vi "Retroespalhamento.vi"() -> ()   [LabVIEW 2019]
uses:
  <vilib>/Analysis/4window.llb/windowTd.ctl
  <vilib>/Analysis/baseanly.llb/Mean (DBL).vi
  <vilib>/Waveform/WDTOps.llb/WDT Number of Waveform Samples DBL.vi
  <vilib>/Waveform/WDTOps.llb/WDT Get Waveform Subset DBL (LV80).vi
  Agilent 6000 Series/Public/Data/Read Single Waveform.vi
  <vilib>/measure/maspectr.llb/FFT Power Spectral Density for 1 Chan.vi
  Instance           2 25Saved   Retroespalhamento .vi
  Instance           4 25Saved   Retroespalhamento .vi
  Instance           3 25Saved   Retroespalhamento .vi
  <vilib>/Analysis/NI_AALPro.lvlib
  Agilent 2000 3000 X-Series/Agilent 2000 3000 X-Series.lvlib
  Agilent 6000 Series/Agilent 6000 Series.lvlib
  <vilib>/measure/NI_MABase.lvlib
  <vilib>/gmath/NI_Gmath.lvlib
  <vilib>/measure/NI_MAPro.lvlib
  <vilib>/Analysis/NI_AALBase.lvlib
panel:
  in  "Freq":dbl
  in  "N of Sample":dbl
  out "Valores do Arquivo TXT":i32[](array[numeric])
  out "output cluster":T1
  out "dfnovo":dbl
  out "FFT1":waveform(dbl)(graph)
  out "FFT2":waveform(dbl)(graph)
  out "df 2":dbl
  out "Espectro novo":dbl[](array[numeric]) format="%_6g"
  in  "Observações":string
  in  "Jump Button":bool
  in  "Save Button":bool
  out "refnum out":refnum<file>
  in  "Repetição":u16(ring) items=["Repetição 1", "Repetição 2", "Repetição 3", "Repetição 4"]
  out "Tabela de Resultados":string[][](table)=[["Repetição ", "AIB", "FSAB", "TSAB"], ["1", "0", "0", "0"], ["2", "0", "0", "0"], ["3", "0", "0", "0"], ["4", "0", "0", "0"]]
  out "TSAB":dbl format="%#_3g"
  in  "Play Button 2":bool
  out "TSAB":dynamicdata(graph)
  out "AIB's":dbl[](array[numeric])
  out "Freq. central":dbl format="%#_3g"
  out "FSAB":dbl format="%#_3g"
  out "size(s)":i32
  out "AIB":dbl format="%#_5g"
  out "Fmax":dbl format="%#_3g"
  out "Fmin":dbl format="%#_3g"
  out "df":dbl
  out "dt":dbl
  in  "Filename":path=path "test.lvm"
  out "FSAB":dynamicdata(graph)
  out "ABTF":waveform(dbl)(graph)
  out "ABTF":dbl[](array[numeric])
  in  "Play Button":bool
  in  "method 4":u16(ring) items=["Least Square", "Least Absolute Residual", "Bisquare"]
  out "Espectro osso":dbl[](array[numeric])
  in  "Captura 2":bool
  in  "Captura":bool
  in  "Parar":bool
  out "Espectro referência":dbl[](array[numeric])
  in  "Quantidade de Capturas":dbl
  out "Waveform com osso":waveform(dbl)(graph)
  in  "method 3":u16(ring) items=["Least Square", "Least Absolute Residual", "Bisquare"]
  in  "Signal Conditioning?":bool
  out "Waveform Referência":waveform(dbl)(graph)
  in  "Maximum Time (10000 ms)":u32
  in  "VISA":refnum<visa-resource-name>
  in  "Channel":u16(ring) items=["Channel 1", "Channel 2", "Channel 3", "Channel 4"]
  in  "Osciloscópio":u16(ring)=4 items=["DSO 3024A", "DSO 6032A", "Simulation", "Data PEB", "Data Labus", "Choose a Scope"]
  # "Resultados (Résultats)"
  # "Osso (Os)"
  # "Cálculos (Calculs)"
  # "Referência (Référence)"
  # "Configurações"
  # "Osciloscópio"
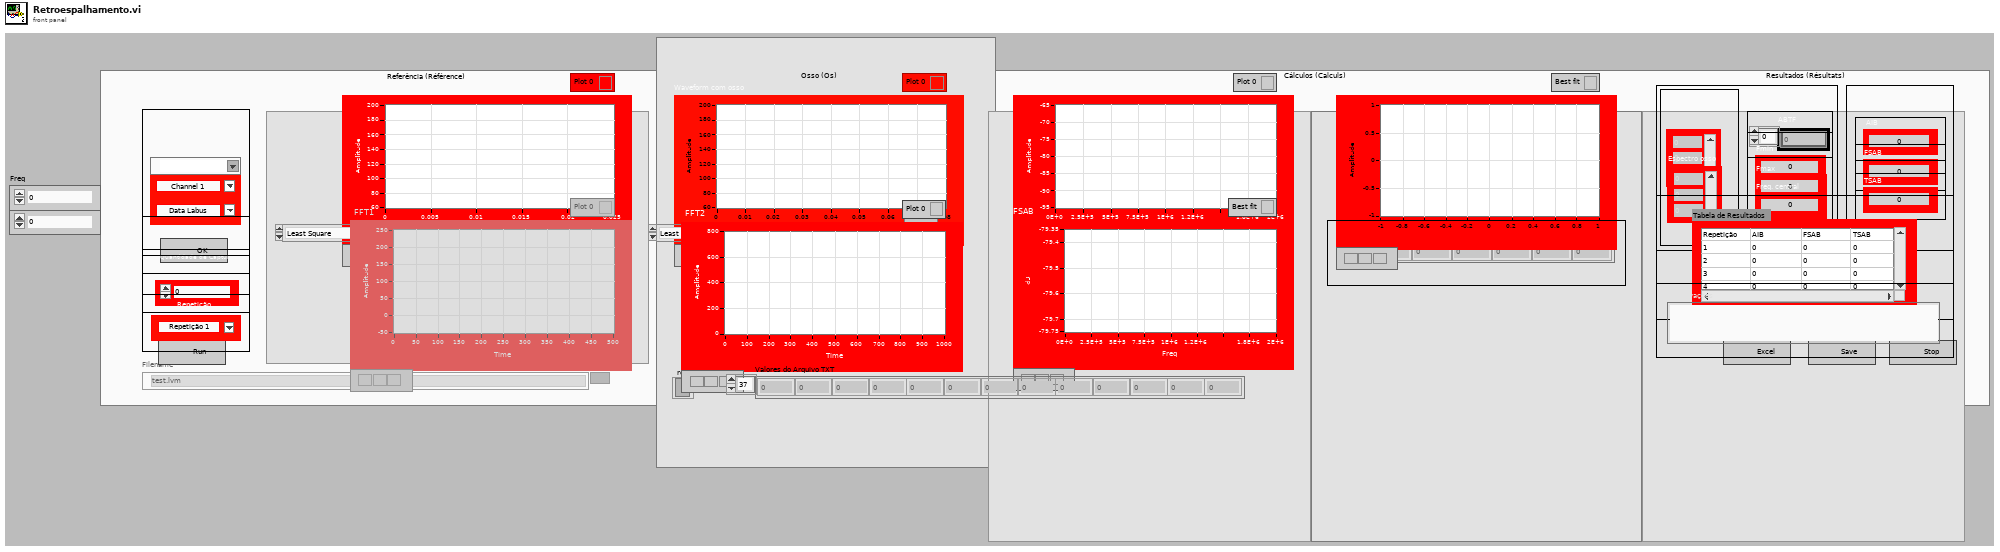
[diagram p1: front panel]
types:
  T1 = cluster{"Waveform Referência":waveform(dbl), "Waveform com osso":waveform(dbl), " FFT1":waveform(dbl), " FFT2":waveform(dbl), "FSAB":dynamicdata, " ABTF":waveform(dbl), "TSAB":dynamicdata, "Tabela de Resultados":string[][], "AIB":dbl, "Fmin":dbl, "Fmax":dbl, "AIB's":dbl[], "TSAB":dbl, "FSAB":dbl, "Observações":string}
  T2 = enum16{"Sine Wave", "Triangle Wave", "Square Wave", "Sawtooth Wave"}
  T3 = enum8{"Enabled", "Disabled", "Disabled and Grayed Out"}
  T4 = typedef "NI_AALPro.lvlib/windowTd.ctl" = u32
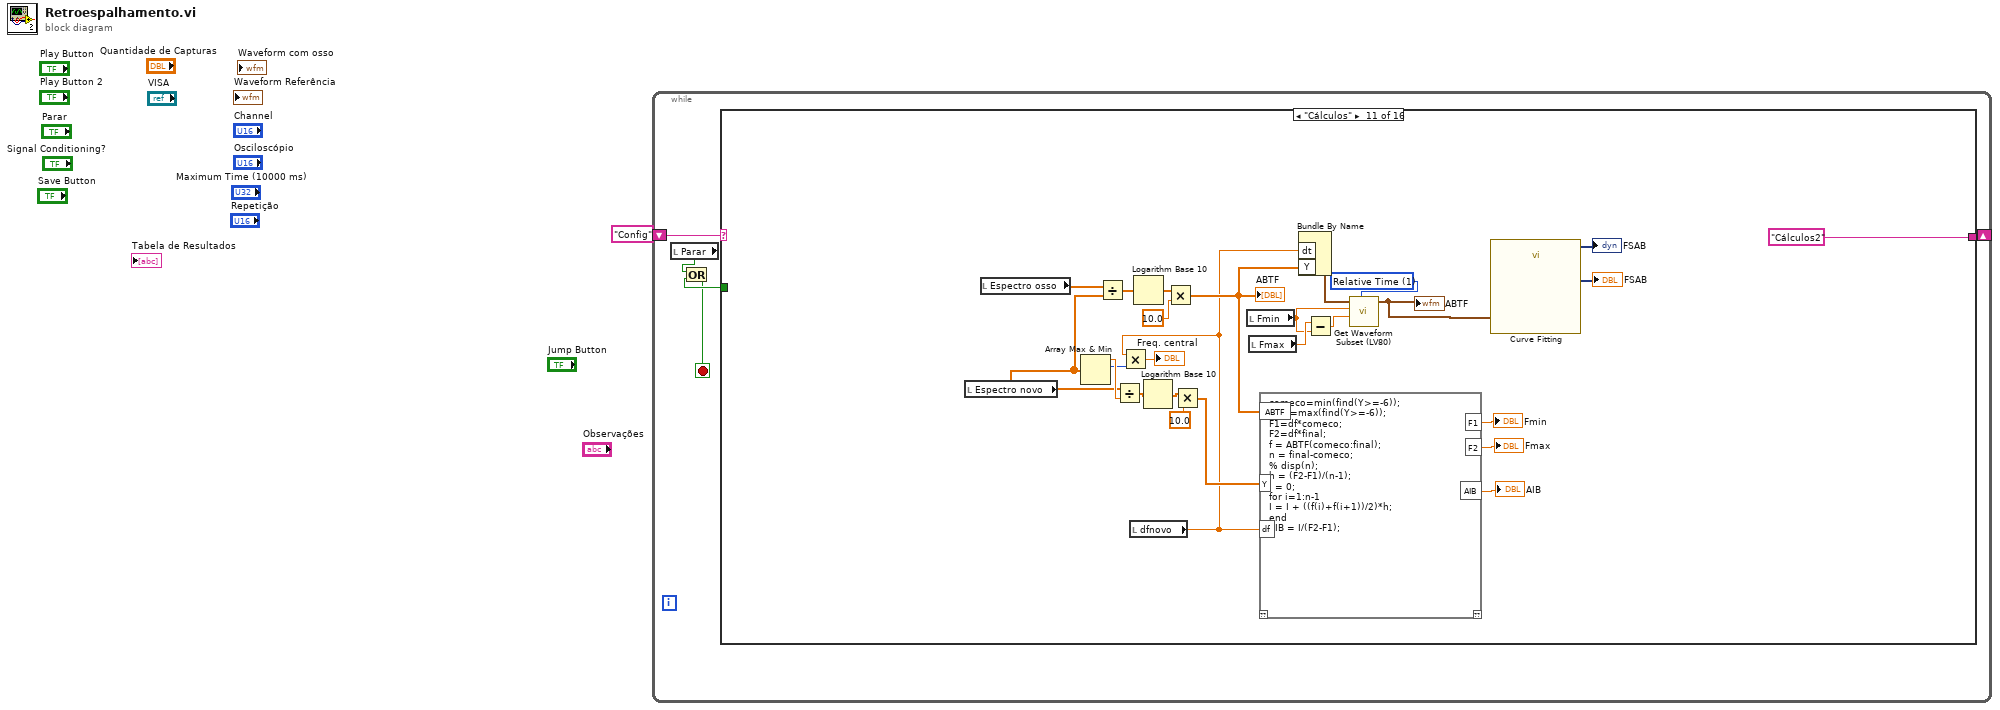
[diagram p0: block diagram]
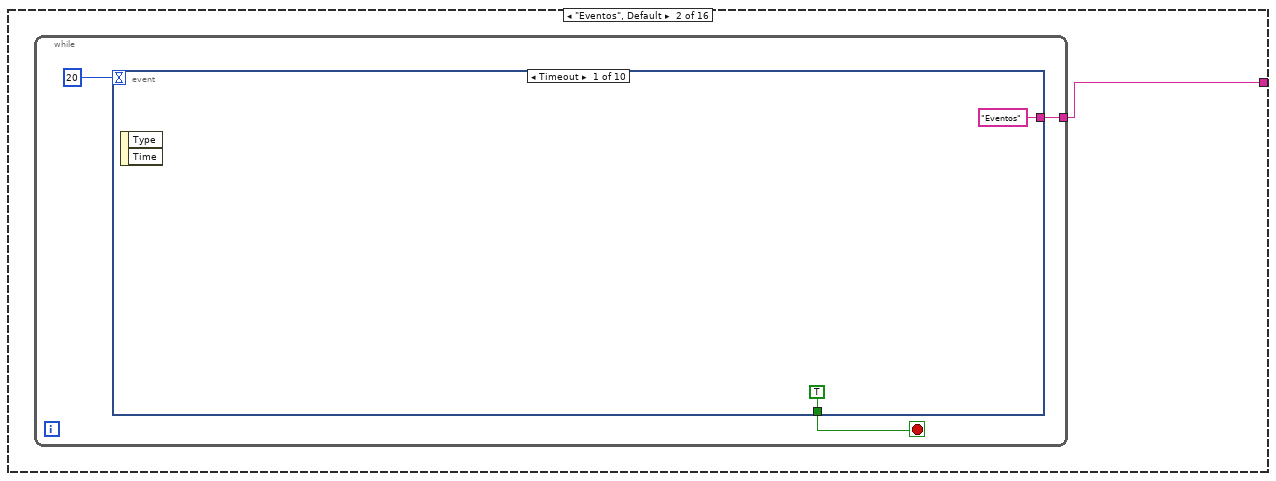
[diagram p3: hidden frame]
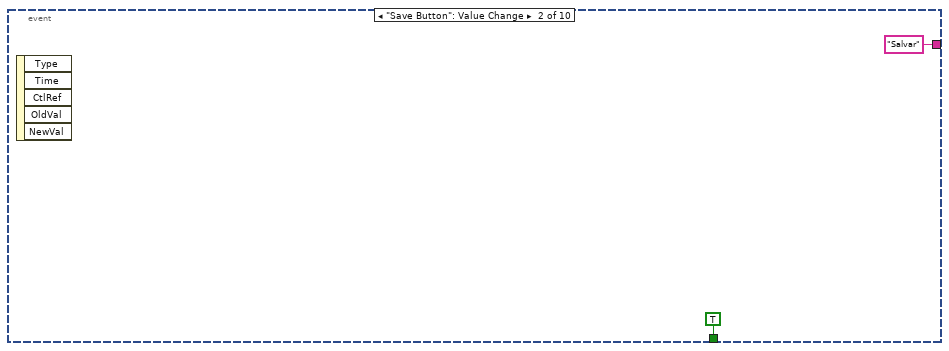
[diagram p4: hidden frame]
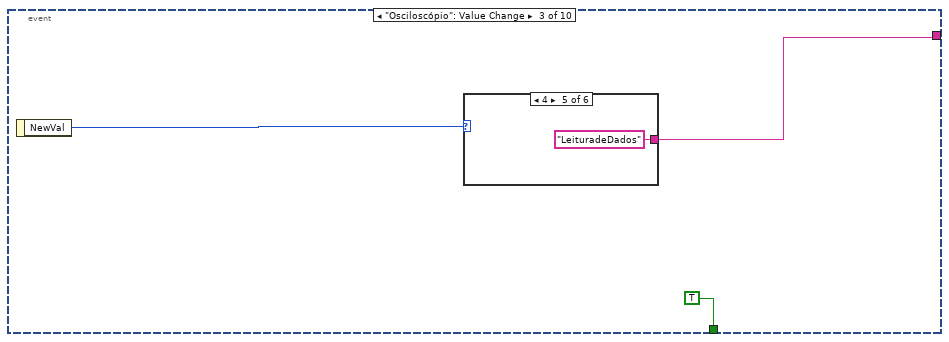
[diagram p5: hidden frame]
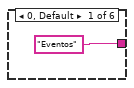
[diagram p6: hidden frame]
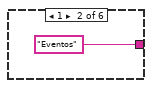
[diagram p7: hidden frame]
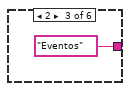
[diagram p8: hidden frame]
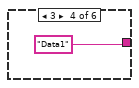
[diagram p9: hidden frame]
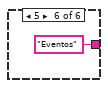
[diagram p10: hidden frame]
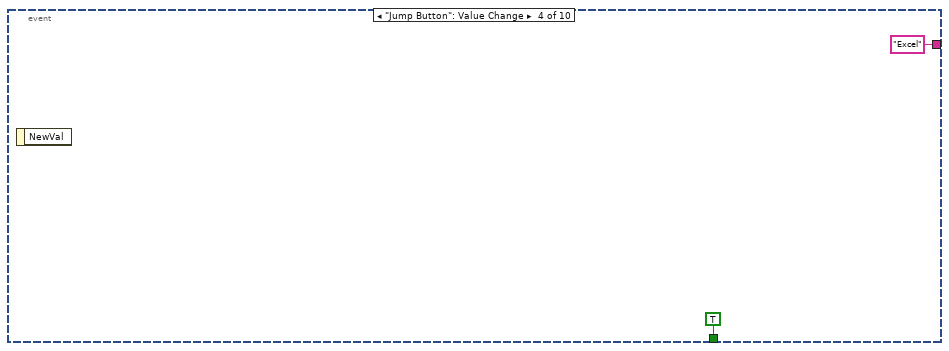
[diagram p11: hidden frame]
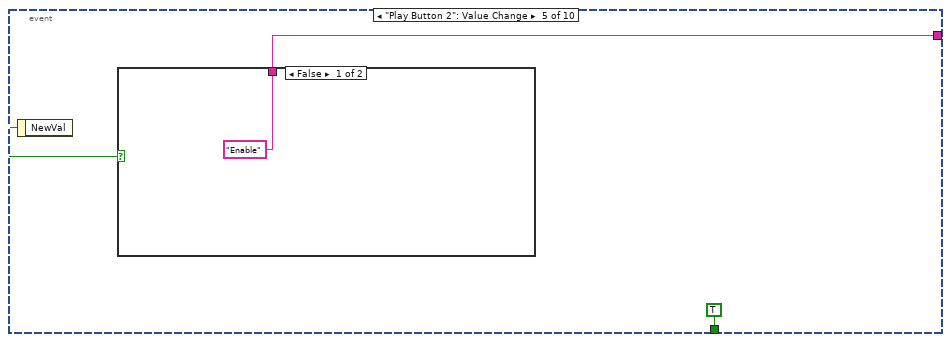
[diagram p12: hidden frame]
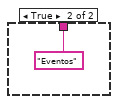
[diagram p13: hidden frame]
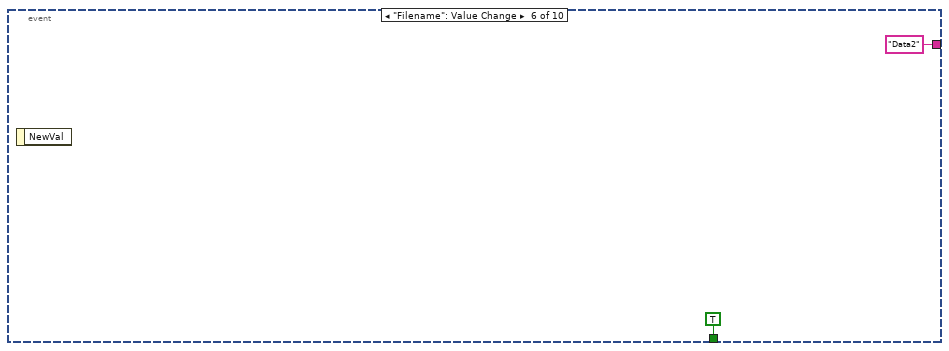
[diagram p14: hidden frame]
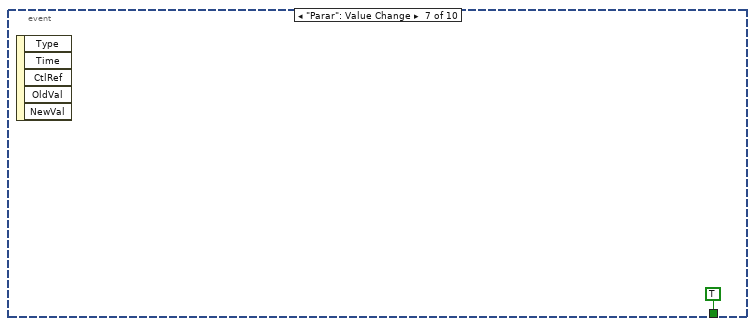
[diagram p15: hidden frame]
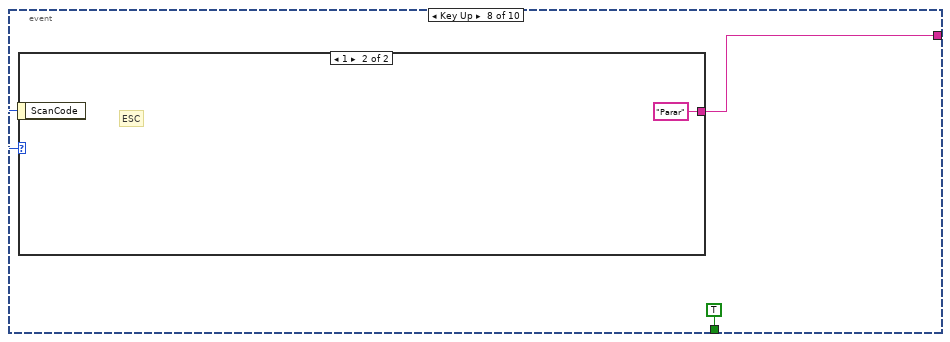
[diagram p16: hidden frame]
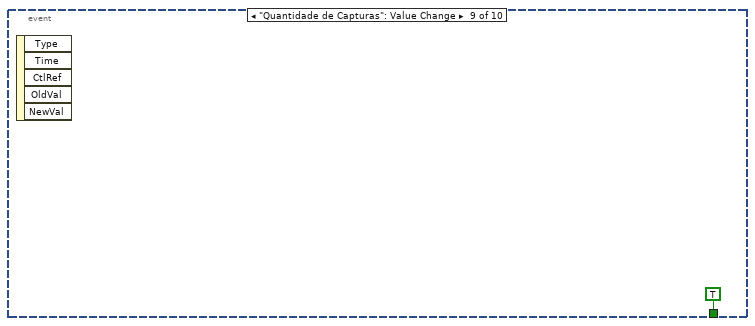
[diagram p18: hidden frame]
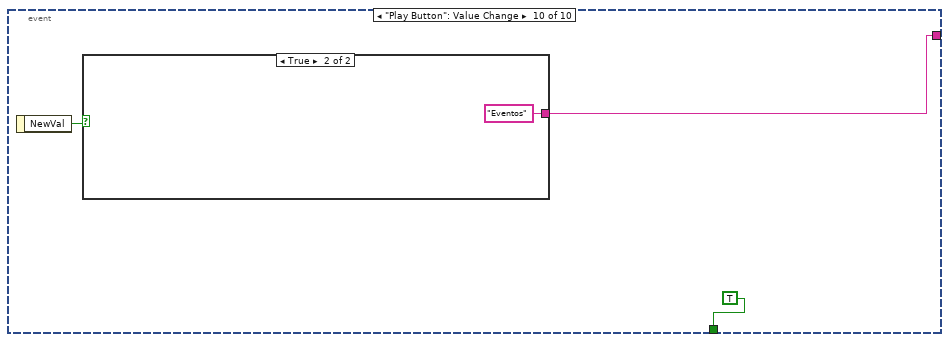
[diagram p19: hidden frame]
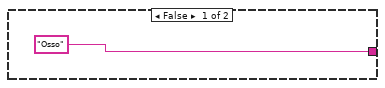
[diagram p20: hidden frame]
diagram:
  n1 = while {
    shift-right: [w5] -> _
    shift-left: "Config" -> [w6]
    stop <- w2 stop-if-true
    n2 = local read "Parar"() -> (w4:bool)
    n3 = case shown="\"Cálculos\"" w6 {
      tunnel: [_ w7 "Referência" "Eventos" "Play" "Eventos" "Eventos" "Cálculos" "Cálculos" _ "Cálculos2" "Tabela" "Eventos" "Eventos" _ "Eventos"] -> w5
      tunnel: [_ _ _ _ FALSE _ _ _ _ TRUE _ _ _ _ _ _] -> w3
      frame "0" {
      }
      frame "Eventos", Default {
        n4 = while {
          tunnel: [w8] -> w7
          stop <- w9 stop-if-true
          n5 = event shown="[0] Timeout" {
            selector: _ -> [_ _ _ _ _ _ _ _ _ _]
            dyn-events: _ -> [_ _ _ _ _ _ _ _ _ _]
            timeout: 20 -> [_ _ _ _ _ _ _ _ _ _]
            tunnel: [TRUE TRUE TRUE TRUE TRUE TRUE TRUE TRUE TRUE TRUE] -> w9
            tunnel: ["Eventos" "Salvar" w15 "Excel" w26 "Data2" _ w35 _ w39] -> w8
            event Timeout {
              n6 = event-data() -> ()  [unwired: 1 in, 2 out]
            }
            event "Save Button": Value Change {
              n7 = event-data() -> ()  [unwired: 1 in, 5 out]
            }
            event "Osciloscópio": Value Change {
              n8 = event-data() -> ("NewVal"=w16:u16)  [unwired: 1 in]
              n9 = case shown="4" w16 {
                tunnel: ["Eventos" "Eventos" "Eventos" "Data1" "LeituradeDados" "Eventos"] -> w15
                frame 0, Default {
                }
                frame 1 {
                }
                frame 2 {
                }
                frame 3 {
                }
                frame 4 {
                }
                frame 5 {
                }
              }
            }
            event "Jump Button": Value Change {
              n10 = event-data() -> ()  [unwired: 1 in, 1 out]
            }
            event "Play Button 2": Value Change {
              n11 = event-data() -> ("NewVal"=w27:bool)  [unwired: 1 in]
              n12 = case shown="False" w27 {
                tunnel: ["Enable" "Eventos"] -> w26
                frame False {
                }
                frame True {
                }
              }
            }
            event "Filename": Value Change {
              n13 = event-data() -> ()  [unwired: 1 in, 1 out]
            }
            event "Parar": Value Change {
              n14 = event-data() -> ()  [unwired: 1 in, 5 out]
            }
            event Key Up {
              n15 = event-data() -> ("ScanCode"=w36:i16)  [unwired: 1 in]
              n16 = case shown="1" w36 {
                tunnel: [_ "Parar"] -> w35
                frame 0, Default {
                }
                frame 1 {
                  # "ESC"
                }
              }
            }
            event "Quantidade de Capturas": Value Change {
              n17 = event-data() -> ()  [unwired: 1 in, 5 out]
            }
            event "Play Button": Value Change {
              n18 = event-data() -> ("NewVal"=w40:bool)  [unwired: 1 in]
              n19 = case shown="True" w40 {
                tunnel: ["Osso" "Eventos"] -> w39
                frame False {
                }
                frame True {
                }
              }
            }
          }
        }
      }
      frame "Enable" {
        w44 = T3."Enabled" ("Disabled")
        n20 = property on="Waveform Referência" class="WFGraph (strict)"("DisabledEnum"=w44) -> ()  [unwired: 2 in, 2 out]
        n21 = property on="Captura" class="Bool (strict)"("DisabledEnum"=w44) -> ()  [unwired: 2 in, 2 out]
        n22 = property on="FFT1" class="WFGraph (strict)"("DisabledEnum"=w44) -> ()  [unwired: 2 in, 2 out]
      }
      frame "Config" {
        w47 = u32 9868950
        w46 = T3."Disabled and Grayed Out" ("Disabled")
        n23 = property on="Osciloscópio" class="Ring (strict)"("Val(Sgnl)"=u16 5 ("Value (Signaling)")) -> ()  [unwired: 2 in, 2 out]
        n24 = property on="Play Button" class="Bool (strict)"("DisabledEnum"=w46) -> ()  [unwired: 2 in, 2 out]
        n25 = property on="Filename" class="Path"("DisabledEnum"=w46) -> ()  [unwired: 2 in, 2 out]
        n26 = property on="Captura 2" class="Bool (strict)"("DisabledEnum"=w46) -> ()  [unwired: 2 in, 2 out]
        n27 = property on="Waveform Referência" class="WFGraph (strict)"("DisabledEnum"=w46) -> ()  [unwired: 2 in, 2 out]
        n28 = property on="FFT1" class="WFGraph (strict)"("DisabledEnum"=w46) -> ()  [unwired: 2 in, 2 out]
        n29 = property on="Captura" class="Bool (strict)"("DisabledEnum"=w46) -> ()  [unwired: 2 in, 2 out]
        n30 = property on="Waveform com osso" class="WFGraph (strict)"("DisabledEnum"=w46) -> ()  [unwired: 2 in, 2 out]
        n31 = property on="FFT2" class="WFGraph (strict)"("DisabledEnum"=w46) -> ()  [unwired: 2 in, 2 out]
        n32 = property on="Channel" class="Ring (strict)"("Strings []"=string[] ["Channel 1", "Channel 2", "Channel 3", "Channel 4"]) -> ()  [unwired: 2 in, 2 out]
        n33 = property on="Repetição" class="Ring (strict)"("Strings []"=string[] ["Repetição 1", "Repetição 2", "Repetição 3", "Repetição 4"]) -> ()  [unwired: 2 in, 2 out]
        n34 = property on="Osciloscópio" class="Ring (strict)"("Strings []"=string[] ["DSO 3024A", "DSO 6032A", "Simulation", "Data PEB", "Data Labus", "Choose a Scope"]) -> ()  [unwired: 2 in, 2 out]
        n35 = while {
          stop <- w65 stop-if-true
          n36 = One Button Dialog(message="Ajustar a caixa \"Configurações\" e clicar em \"Run\"", button name ("OK")="Ok") -> (true=w65:bool)
        }
        n37 = property on="Tabela de Resultados" class="Tbl (strict)"("Value"=string[][] [["Repetição ", "AIB", "FSAB", "TSAB"], ["1", "0", "0", "0"], ["2", "0", "0", "0"], ["3", "0", "0", "0"], ["4", "0", "0", "0"]] ("Table Control"), "Number of Columns"=u32 4, "Number of Rows"=u32 5, "Cell BG Color"=w47, "Active Cell"=cluster{"Row":i32, "Column":i32} {"Row"=0, "Column"=1} ("Active Cell:Active Cell"), "Cell BG Color"=w47, "Active Cell"=cluster{"Row":i32, "Column":i32} {"Row"=0, "Column"=2} ("Active Cell:Active Cell"), "Cell BG Color"=w47, "Active Cell"=cluster{"Row":i32, "Column":i32} {"Row"=0, "Column"=3} ("Active Cell:Active Cell"), "Cell BG Color"=w47, "Active Cell"=cluster{"Row":i32, "Column":i32} {"Row"=1, "Column"=0} ("Active Cell:Active Cell"), "Cell BG Color"=w47, "Active Cell"=cluster{"Row":i32, "Column":i32} {"Row"=2, "Column"=0} ("Active Cell:Active Cell"), "Cell BG Color"=w47, "Active Cell"=cluster{"Row":i32, "Column":i32} {"Row"=3, "Column"=0} ("Active Cell:Active Cell"), "Cell BG Color"=w47, "Active Cell"=cluster{"Row":i32, "Column":i32} {"Row"=4, "Column"=0} ("Active Cell:Active Cell"), "Cell BG Color"=w47) -> ()  [unwired: 2 in, 2 out]
      }
      frame "Referência" {
        w81 = 2 items=["nearest", "linear", "spline", "cubic Hermite", "Lagrange"] ("method")
        w90 = u16 1 items=["Samples", "Relative Time"] ("start/duration format")
        n38 = property on="Osciloscópio" class="Ring (strict)"() -> ("Value"=w94:u16)  [unwired: 2 in, 2 out]
        n39 = local read "VISA"() -> (w96:refnum<visa-resource-name>)
        n40 = local read "Maximum Time (10000 ms)"() -> (w95:u32)
        n41 = property on="Channel" class="Ring (strict)"() -> ("Value"=w97:u16)  [unwired: 2 in, 2 out]
        n42 = while {
          tunnel: w97 -> [w117]
          tunnel: w96 -> [w116]
          tunnel: w95 -> [w115]
          tunnel: w94 -> [w113]
          tunnel: [w107] -> w92
          tunnel: [w104] -> w85
          tunnel: [w103] -> w86
          stop <- "Captura" stop-if-true
          n43 = case shown="0" w113 {
            tunnel: [w130 w142 w159] -> w108
            tunnel: w117 -> [w132 w141 _]
            tunnel: w116 -> [w134 w140 _]
            tunnel: w115 -> [_ _ _]
            frame 0 {
              w129 = u16 0 items=["Samples", "Relative Time"] ("start/duration format")
              n44 = Wait Until Next ms Multiple(millisecond multiple=u32 10) -> ()  [unwired: 1 out]
              n45 = call-poly "Read Waveforms.vi"("Source Channel (0: Channel 1)"=w132, "VISA resource name"=w134) -> ("error out"=w133:errorcluster, "Waveform Data"=w128:waveform(dbl), "VISA resource name out"=w135:refnum<visa-resource-name>)  [unwired: 7 in]
              n46 = call-poly <vilib>:"Number of Waveform Samples.vi"("waveform in"=w128) -> ("number of samples"=w136:i32)  [unwired: 8 in, 2 out]
              n47 = Decrement(x=w136) -> (x-1=w137:i32)
              n48 = To Double Precision Float(number=w137) -> (double precision float=w131:dbl)
              n49 = call "Close.vi"("error in (no error)"=w133, "VISA resource name"=w135) -> ("error out"=w138:errorcluster)  [unwired: 9 out]
              n50 = call-poly <vilib>:"Get Waveform Subset (LV80).vi"("start/duration format"=w129, "duration"=w131, "waveform in"=w128) -> ("waveform out"=w130:waveform(dbl))  [unwired: 3 in, 3 out]
              n51 = call <vilib>:"Simple Error Handler.vi"("error in (no error)"=w138) -> ()  [unwired: 1 in, 8 out]
            }
            frame 1, Default {
              w147 = FALSE ("Reset? (T: Yes)")
              n52 = call "Initialize.vi"("Reset? (T: Yes)"=w147, "ID Query? (T: Yes)"=w147, "VISA resource name"=w140) -> ("error out"=w145:errorcluster, "VISA resource name out"=w146:refnum<visa-resource-name>)  [unwired: 7 in]
              n53 = call-poly "Read.vi"("error in (no error)"=w145, "Timeout (10000 ms)"=u32 10000, "Source (0: Channel 1)"=w141, "VISA resource name"=w146) -> ("error out"=w148:errorcluster, "Waveform Data"=w142:waveform(dbl), "VISA resource name out"=w149:refnum<visa-resource-name>)  [unwired: 5 in]
              n54 = call "Close.vi"("error in (no error)"=w148, "VISA resource name"=w149) -> ("error out"=w150:errorcluster)  [unwired: 9 in]
              n55 = Wait Until Next ms Multiple(millisecond multiple=u32 10) -> ()  [unwired: 1 out]
              n56 = call <vilib>:"Simple Error Handler.vi"("error in (no error)"=w150) -> ()  [unwired: 4 in, 5 out]
            }
            frame 2 {
              w152 = 10.0 ("y")
              w151 = 5.0 ("y")
              n57 = Random Number (0-1)() -> (number: 0 to 1=w155:dbl)
              n58 = Random Number (0-1)() -> (number: 0 to 1=w158:dbl)
              n59 = Increment(x=w155) -> (x+1=w156:dbl)
              n60 = Increment(x=w158) -> (x+1=w157:dbl)
              n61 = Multiply(x=w156, y=w152) -> ()  [unwired: 1 out]
              n62 = Multiply(x=w157, y=w151) -> ()  [unwired: 1 out]
              n63 = call <vilib>:"Basic Function Generator.vi"("signal type"=T2."Sine Wave", "amplitude"=w152, "frequency"=w151) -> ("signal out"=w159:waveform(dbl))  [unwired: 6 in, 2 out]
              n64 = Wait (ms)(milliseconds to wait=u32 200) -> ()  [unwired: 1 out]
            }
          }
          n65 = local read "Signal Conditioning?"() -> (w112:bool)
          n66 = Unbundle By Name(w108) -> ("dt"=w111:dbl, "Y"=w110:dbl[])
          n67 = property on="Waveform Referência" class="WFGraph (strict)"("Active Cursor"=u32 0, "Active Cursor"=u32 1) -> ("Cursor.Cursor X"=w104:dbl, "Cursor.Cursor X"=w103:dbl)  [unwired: 2 in, 2 out]
          n68 = case shown="True" w112 {
            tunnel: [w118 w119] -> w109
            tunnel: w110 -> [w118 w121]
            tunnel: w111 -> [_ w120]
            frame False {
            }
            frame True {
              n69 = Array Size(array=w121) -> (size(s)=w126:i32)
              n70 = for {
                N: w126 -> [_]
                tunnel: [w127] -> w125 mode=indexing
                i -> [w127]
              }
              n71 = Multiply(x=w120, y=w125) -> (x*y=w124:dbl[])
              n72 = call <vilib>:"General Polynomial Fit.vi"("Y"=w121, "X"=w124, "algorithm"="method 3") -> ("Best Polynomial Fit"=w123:dbl[])  [unwired: 9 in, 3 out]
              n73 = Subtract(x=w121, y=w123) -> (x-y=w119:dbl[])
            }
          }
          n74 = Bundle By Name(cluster=w108, "Y"=w109) -> (w107:waveform(dbl))
          n75 = local write "Waveform Referência"(w107) -> ()
        }
        n76 = local read "df"() -> (w67:dbl)
        n77 = Subtract(x=w86, y=w85) -> (x-y=w87:dbl)
        n78 = call-poly <vilib>:"Get Waveform Subset (LV80).vi"("start/duration format"=w90, "duration"=w87, "start samples/time"=w85, "waveform in"=w92) -> ("error out"=w82:errorcluster, "waveform out"=w84:waveform(dbl))  [unwired: 2 in, 2 out]
        n79 = call-poly <vilib>:"FFT Power Spectral Density.vi"("error in (no error)"=w82, "dB On (F)"=FALSE, "time signal"=w84) -> ("power spectral density"=w83:cluster{"f0":dbl, "df":dbl, "magnitude":dbl[]})  [unwired: 5 in, 3 out]
        n80 = local write "Waveform Referência"(w84) -> ()
        n81 = Unbundle By Name(w83) -> ("magnitude"=w68:dbl[], "df"=w89:dbl)
        "Espectro referência" <- w68
        n82 = Array Size(array=w68) -> (size(s)=w78:i32)
        n83 = Initialize Array(0.0 ("element"), w78) -> (w79:dbl[])
        n84 = for {
          N: w78 -> [_]
          shift-right: [w101] -> w77
          shift-left: w79 -> [w102]
          tunnel: w67 -> [w99]
          i -> [w100]
          n85 = Multiply(x=w99, y=w100) -> (x*y=w98:dbl)
          n86 = Replace Array Subset(array=w102, new element=w98, index=w100) -> (w101:dbl[])
        }
        n87 = call <vilib>:"Interpolate 1D.vi"("ntimes"=4, "method"=w81, "X"=w77, "Y"=w68) -> ("xi used"=w75:dbl[], "yi"=w66:dbl[])  [unwired: 5 in, 1 out]
        "Espectro novo" <- w66
        n88 = Index Array(array=w75, index=2) -> (element=w72:dbl)
        n89 = Index Array(array=w75, index=1) -> (element=w71:dbl)
        n90 = Subtract(x=w72, y=w71) -> (x-y=w70:dbl)
        "dfnovo" <- w70
        n91 = Bundle By Name("dt"=w70, "Y"=w66) -> (→"FFT1":waveform(dbl))  [unwired: 1 in]
        n92 = local write "df"(w89) -> ()
      }
      frame "Play" {
        w160 = T3."Enabled" ("Disabled")
        n93 = property on="FFT2" class="WFGraph (strict)"("DisabledEnum"=w160) -> ()  [unwired: 2 in, 2 out]
        n94 = property on="Captura 2" class="Bool (strict)"("DisabledEnum"=w160) -> ()  [unwired: 2 in, 2 out]
        n95 = property on="Waveform com osso" class="WFGraph (strict)"("DisabledEnum"=w160) -> ()  [unwired: 2 in, 2 out]
        n96 = property on="Play Button" class="Bool (strict)"("DisabledEnum"=w160) -> ()  [unwired: 2 in, 2 out]
        n97 = while {
          stop <- w162 stop-if-true
          n98 = One Button Dialog(message="Posicione o osso no refletor e clique em \"Play\" para começar a medição ou clique em \"Run\" para refazer a medição do refletor", button name ("OK")="Ok") -> (true=w162:bool)
        }
      }
      frame "Data1" {
        w190 = 2 items=["nearest", "linear", "spline", "cubic Hermite", "Lagrange"] ("method")
        w192 = T3."Enabled" ("Disabled")
        w196 = u16 1 items=["Samples", "Relative Time"] ("start/duration format")
        n99 = local read "N of Sample"() -> (w170:dbl)
        n100 = property on="Filename" class="Path"("DisabledEnum"=w192) -> ()  [unwired: 2 in, 2 out]
        n101 = property on="Captura" class="Bool (strict)"("DisabledEnum"=w192) -> ()  [unwired: 2 in, 2 out]
        n102 = property on="Waveform Referência" class="WFGraph (strict)"("DisabledEnum"=w192) -> ()  [unwired: 2 in, 2 out]
        n103 = property on="FFT1" class="WFGraph (strict)"("DisabledEnum"=w192) -> ()  [unwired: 2 in, 2 out]
        n104 = Read from Text File(file (use dialog)="Filename") -> (text=w174:string)  [unwired: 3 in, 3 out]
        n105 = Decrement(x=w170) -> (x-1=w172:dbl)
        n106 = for {
          N: w172 -> [_]
          tunnel: w174 -> [w206]
          tunnel: [w205] -> w171 mode=indexing
          shift-right: [w202] -> _
          shift-left: 0 -> [w203]
          n107 = Fract/Exp String To Number(string=w206, offset=w203) -> (number=w205:dbl)  [unwired: 2 in, 1 out]
          n108 = Add(x=w203, y=4.0) -> (x+y=w202:dbl)
        }
        "Valores do Arquivo TXT" <- w171
        n109 = Divide(x="N of Sample", y="Freq") -> (x/y=w169:dbl)
        n110 = Bundle By Name("Y"=w171, "dt"=w169) -> (w165:waveform(dbl))  [unwired: 1 in]
        n111 = while {
          tunnel: [w215] -> w199
          tunnel: [w214] -> w198
          tunnel: w165 -> [w213]
          stop <- w212 stop-if-true
          n112 = local write "Waveform Referência"(w213) -> ()
          n113 = property on="Waveform Referência" class="WFGraph (strict)"("Active Cursor"=u32 0, "Active Cursor"=u32 1) -> ("Cursor.Cursor X"=w214:dbl, "Cursor.Cursor X"=w215:dbl)  [unwired: 2 in, 2 out]
          n114 = local read "Captura"() -> (w212:bool)
        }
        n115 = local read "df"() -> (w177:dbl)
        n116 = Subtract(x=w199, y=w198) -> (x-y=w197:dbl)
        n117 = call-poly <vilib>:"Get Waveform Subset (LV80).vi"("start/duration format"=w196, "duration"=w197, "start samples/time"=w198, "waveform in"=w165) -> ("waveform out"=w193:waveform(dbl))  [unwired: 2 in, 3 out]
        n118 = local write "Waveform Referência"(w193) -> ()
        n119 = Unbundle By Name(w193) -> ("dt"=→"dt":dbl)  [unwired: 1 out]
        n120 = call-poly <vilib>:"FFT Power Spectral Density.vi"("dB On (F)"=FALSE, "time signal"=w193) -> ("power spectral density"=w201:cluster{"f0":dbl, "df":dbl, "magnitude":dbl[]})  [unwired: 6 in, 3 out]
        n121 = Unbundle By Name(w201) -> ("magnitude"=w178:dbl[], "df"=→"df":dbl)
        n122 = Array Size(array=w178) -> (size(s)=w187:i32)
        n123 = Initialize Array(0.0 ("element"), w187) -> (w188:dbl[])
        n124 = for {
          N: w187 -> [_]
          shift-right: [w210] -> w186
          shift-left: w188 -> [w211]
          tunnel: w177 -> [w208]
          i -> [w209]
          n125 = Multiply(x=w208, y=w209) -> (x*y=w207:dbl)
          n126 = Replace Array Subset(array=w211, new element=w207, index=w209) -> (w210:dbl[])
        }
        n127 = local write "Espectro referência"(w178) -> ()
        n128 = call <vilib>:"Interpolate 1D.vi"("ntimes"=4, "method"=w190, "X"=w186, "Y"=w178) -> ("xi used"=w184:dbl[], "yi"=w176:dbl[])  [unwired: 5 in, 1 out]
        n129 = Index Array(array=w184, index=2) -> (element=w181:dbl)
        n130 = Index Array(array=w184, index=1) -> (element=w180:dbl)
        n131 = Subtract(x=w181, y=w180) -> (x-y=w175:dbl)
        n132 = Bundle By Name("dt"=w175, "Y"=w176) -> (w179:waveform(dbl))  [unwired: 1 in]
        n133 = local write "Espectro novo"(w176) -> ()
        n134 = local write "dfnovo"(w175) -> ()
        n135 = local write "FFT1"(w179) -> ()
      }
      frame "Data2" {
        w231 = u16 0 items=["Samples", "Relative Time"] ("start/duration format")
        w236 = T3."Enabled" ("Disabled")
        w238 = u16 1 items=["Samples", "Relative Time"] ("start/duration format")
        n136 = local read "Filename"() -> (w222:path)
        n137 = local read "N of Sample"() -> (w224:dbl)
        n138 = property on="Captura 2" class="Bool (strict)"("DisabledEnum"=w236) -> ()  [unwired: 2 in, 2 out]
        n139 = property on="Waveform com osso" class="WFGraph (strict)"("DisabledEnum"=w236) -> ()  [unwired: 2 in, 2 out]
        n140 = property on="FFT2" class="WFGraph (strict)"("DisabledEnum"=w236) -> ()  [unwired: 2 in, 2 out]
        n141 = local read "Freq"() -> (w219:dbl)
        n142 = Read from Text File(file (use dialog)=w222) -> (text=w227:string)  [unwired: 3 in, 3 out]
        n143 = Decrement(x=w224) -> (x-1=w225:dbl)
        n144 = for {
          N: w225 -> [_]
          tunnel: w227 -> [w249]
          tunnel: [w248] -> w218 mode=indexing
          shift-right: [w245] -> _
          shift-left: 0 -> [w246]
          n145 = Fract/Exp String To Number(string=w249, offset=w246) -> (number=w248:dbl)  [unwired: 2 in, 1 out]
          n146 = Add(x=w246, y=4.0) -> (x+y=w245:dbl)
        }
        n147 = local read "N of Sample"() -> (w220:dbl)
        n148 = Divide(x=w220, y=w219) -> (x/y=w223:dbl)
        n149 = Bundle By Name("Y"=w218, "dt"=w223) -> (w221:waveform(dbl))  [unwired: 1 in]
        n150 = local write "Valores do Arquivo TXT"(w218) -> ()
        n151 = while {
          tunnel: [w253] -> w241
          tunnel: [w252] -> w240
          tunnel: w221 -> [w251]
          stop <- w250 stop-if-true
          n152 = local write "Waveform com osso"(w251) -> ()
          n153 = property on="Waveform com osso" class="WFGraph (strict)"("Active Cursor"=u32 0, "Active Cursor"=u32 1) -> ("Cursor.Cursor X"=w252:dbl, "Cursor.Cursor X"=w253:dbl)  [unwired: 2 in, 2 out]
          n154 = local read "Captura 2"() -> (w250:bool)
        }
        n155 = Subtract(x=w241, y=w240) -> (x-y=w239:dbl)
        n156 = call-poly <vilib>:"Get Waveform Subset (LV80).vi"("start/duration format"=w238, "duration"=w239, "start samples/time"=w240, "waveform in"=w221) -> ("waveform out"=w242:waveform(dbl))  [unwired: 2 in, 3 out]
        n157 = local write "Waveform com osso"(w242) -> ()
        n158 = call-poly <vilib>:"FFT Power Spectral Density.vi"("dB On (F)"=FALSE, "time signal"=w242) -> ("power spectral density"=w244:cluster{"f0":dbl, "df":dbl, "magnitude":dbl[]})  [unwired: 6 in, 3 out]
        n159 = Unbundle By Name(w244) -> ("magnitude"=w228:dbl[], "df"=w229:dbl)
        n160 = call-poly <vilib>:"Number of Waveform Samples.vi"("waveform in"=w228) -> ("number of samples"=w233:i32)  [unwired: 8 in, 2 out]
        n161 = Decrement(x=w233) -> (x-1=w234:i32)
        n162 = local write "Espectro osso"(w228) -> ()
        n163 = To Double Precision Float(number=w234) -> (double precision float=w232:dbl)
        n164 = call-poly <vilib>:"Get Waveform Subset (LV80).vi"("start/duration format"=w231, "duration"=w232, "waveform in"=w228) -> ("waveform out"=w230:waveform(dbl))  [unwired: 3 in, 3 out]
        n165 = Bundle By Name("Y"=w230, "dt"=w229) -> (w235:waveform(dbl))  [unwired: 1 in]
        n166 = local write "FFT2"(w235) -> ()
      }
      frame "Osso" {
        w261 = u16 0 items=["Samples", "Relative Time"] ("start/duration format")
        w256 = T3."Enabled" ("Disabled")
        w276 = u16 1 items=["Samples", "Relative Time"] ("start/duration format")
        n167 = local read "Quantidade de Capturas"() -> (w271:dbl)
        n168 = for {
          N: w271 -> [_]
          tunnel: [w286] -> w268 mode=indexing
          tunnel: [w287] -> w273
          tunnel: [w284] -> w270
          tunnel: [w283] -> w269
          n169 = property on="Osciloscópio" class="Ring (strict)"() -> ("Value"=w290:u16)  [unwired: 2 in, 2 out]
          n170 = local read "VISA"() -> (w291:refnum<visa-resource-name>)
          n171 = local read "Maximum Time (10000 ms)"() -> (w289:u32)
          n172 = property on="Channel" class="Ring (strict)"() -> ("Value"=w292:u16)  [unwired: 2 in, 2 out]
          n173 = while {
            tunnel: w292 -> [w307]
            tunnel: w291 -> [w306]
            tunnel: w289 -> [w305]
            tunnel: w290 -> [w304]
            tunnel: [w298] -> w287
            tunnel: [w294] -> w284
            tunnel: [w293] -> w283
            stop <- "Captura 2" stop-if-true
            n174 = case shown="1, Default" w304 {
              tunnel: [w318 w332 w349] -> w299
              tunnel: w307 -> [w324 w331 _]
              tunnel: w306 -> [w325 w330 _]
              tunnel: w305 -> [_ _ _]
              frame 0 {
                w320 = u16 0 items=["Samples", "Relative Time"] ("start/duration format")
                n175 = Wait Until Next ms Multiple(millisecond multiple=u32 10) -> ()  [unwired: 1 out]
                n176 = call "Read Waveforms (Single).vi"("Source Channel (0: Channel 1)"=w324, "VISA resource name"=w325) -> ("error out"=w327:errorcluster, "Waveform Data"=w319:waveform(dbl), "VISA resource name out"=w328:refnum<visa-resource-name>)  [unwired: 7 in]
                n177 = call-poly <vilib>:"Number of Waveform Samples.vi"("waveform in"=w319) -> ("number of samples"=w322:i32)  [unwired: 8 in, 2 out]
                n178 = Decrement(x=w322) -> (x-1=w323:i32)
                n179 = To Double Precision Float(number=w323) -> (double precision float=w321:dbl)
                n180 = call "Close.vi"("error in (no error)"=w327, "VISA resource name"=w328) -> ("error out"=w326:errorcluster)  [unwired: 9 out]
                n181 = call-poly <vilib>:"Get Waveform Subset (LV80).vi"("start/duration format"=w320, "duration"=w321, "waveform in"=w319) -> ("waveform out"=w318:waveform(dbl))  [unwired: 3 in, 3 out]
                n182 = call <vilib>:"Simple Error Handler.vi"("error in (no error)"=w326) -> ()  [unwired: 1 in, 8 out]
              }
              frame 1, Default {
                w337 = FALSE ("Reset? (T: Yes)")
                n183 = call "Initialize.vi"("Reset? (T: Yes)"=w337, "ID Query? (T: Yes)"=w337, "VISA resource name"=w330) -> ("error out"=w335:errorcluster, "VISA resource name out"=w336:refnum<visa-resource-name>)  [unwired: 7 in]
                n184 = call-poly "Read.vi"("error in (no error)"=w335, "Timeout (10000 ms)"=u32 10000, "Source (0: Channel 1)"=w331, "VISA resource name"=w336) -> ("error out"=w338:errorcluster, "Waveform Data"=w332:waveform(dbl), "VISA resource name out"=w339:refnum<visa-resource-name>)  [unwired: 5 in]
                n185 = call "Close.vi"("error in (no error)"=w338, "VISA resource name"=w339) -> ("error out"=w340:errorcluster)  [unwired: 9 in]
                n186 = Wait Until Next ms Multiple(millisecond multiple=u32 10) -> ()  [unwired: 1 out]
                n187 = call <vilib>:"Simple Error Handler.vi"("error in (no error)"=w340) -> ()  [unwired: 4 in, 5 out]
              }
              frame 2 {
                w341 = 11.0 ("y")
                w342 = 6.0 ("y")
                n188 = Random Number (0-1)() -> (number: 0 to 1=w345:dbl)
                n189 = Random Number (0-1)() -> (number: 0 to 1=w348:dbl)
                n190 = Increment(x=w345) -> (x+1=w346:dbl)
                n191 = Increment(x=w348) -> (x+1=w347:dbl)
                n192 = Multiply(x=w346, y=w341) -> ()  [unwired: 1 out]
                n193 = Multiply(x=w347, y=w342) -> ()  [unwired: 1 out]
                n194 = call <vilib>:"Basic Function Generator.vi"("signal type"=T2."Sine Wave", "amplitude"=w341, "frequency"=w342) -> ("signal out"=w349:waveform(dbl))  [unwired: 6 in, 2 out]
                n195 = Wait (ms)(milliseconds to wait=u32 200) -> ()  [unwired: 1 out]
              }
            }
            n196 = local read "Signal Conditioning?"() -> (w303:bool)
            n197 = Unbundle By Name(w299) -> ("dt"=w302:dbl, "Y"=w301:dbl[])
            n198 = case shown="True" w303 {
              tunnel: [w308 w309] -> w300
              tunnel: w301 -> [w308 w311]
              tunnel: w302 -> [_ w310]
              frame False {
              }
              frame True {
                n199 = Array Size(array=w311) -> (size(s)=w316:i32)
                n200 = for {
                  N: w316 -> [_]
                  tunnel: [w317] -> w315 mode=indexing
                  i -> [w317]
                }
                n201 = Multiply(x=w310, y=w315) -> (x*y=w314:dbl[])
                n202 = call <vilib>:"General Polynomial Fit.vi"("Y"=w311, "X"=w314, "algorithm"="method 4") -> ("Best Polynomial Fit"=w313:dbl[])  [unwired: 9 in, 3 out]
                n203 = Subtract(x=w311, y=w313) -> (x-y=w309:dbl[])
              }
            }
            n204 = Bundle By Name(cluster=w299, "Y"=w300) -> (w298:waveform(dbl))
            n205 = local write "Waveform com osso"(w298) -> ()
            n206 = property on="Waveform com osso" class="WFGraph (strict)"("Active Cursor"=u32 0, "Active Cursor"=u32 1) -> ("Cursor.Cursor X"=w294:dbl, "Cursor.Cursor X"=w293:dbl)  [unwired: 2 in, 2 out]
          }
          n207 = Unbundle By Name(w287) -> ("Y"=w286:dbl[])
          n208 = Array Size(array=w286) -> (size(s)=→"size(s)":i32)
          n209 = Wait (ms)(milliseconds to wait=u32 500) -> ()  [unwired: 1 out]
        }
        n210 = property on="Waveform com osso" class="WFGraph (strict)"("DisabledEnum"=w256) -> ()  [unwired: 2 in, 2 out]
        n211 = property on="Captura 2" class="Bool (strict)"("DisabledEnum"=w256) -> ()  [unwired: 2 in, 2 out]
        n212 = property on="Play Button" class="Bool (strict)"("DisabledEnum"=w256) -> ()  [unwired: 2 in, 2 out]
        n213 = property on="FFT2" class="WFGraph (strict)"("DisabledEnum"=w256) -> ()  [unwired: 2 in, 2 out]
        n214 = Transpose 2D Array(2D array=w268) -> (transposed array=w266:dbl[][])
        n215 = for {
          tunnel: w266 -> [w282] mode=indexing
          tunnel: [w281] -> w267 mode=indexing
          n216 = call-poly <vilib>:"Mean.vi"("X"=w282) -> ("mean"=w281:dbl)  [unwired: 1 out]
        }
        n217 = Bundle By Name(cluster=w273, "Y"=w267) -> (w272:waveform(dbl))
        n218 = local write "Waveform com osso"(w272) -> ()
        n219 = local read "df 2"() -> (w257:dbl)
        n220 = Subtract(x=w269, y=w270) -> (x-y=w278:dbl)
        n221 = call-poly <vilib>:"Get Waveform Subset (LV80).vi"("start/duration format"=w276, "duration"=w278, "start samples/time"=w270, "waveform in"=w272) -> ("error out"=w274:errorcluster, "waveform out"=w275:waveform(dbl))  [unwired: 2 in, 2 out]
        n222 = call-poly <vilib>:"FFT Power Spectral Density.vi"("error in (no error)"=w274, "dB On (F)"=FALSE, "time signal"=w275) -> ("power spectral density"=w277:cluster{"f0":dbl, "df":dbl, "magnitude":dbl[]})  [unwired: 5 in, 3 out]
        n223 = local write "Waveform com osso"(w275) -> ()
        n224 = Unbundle By Name(w277) -> ("magnitude"=w258:dbl[], "df"=→"df 2":dbl)
        "Espectro osso" <- w258
        n225 = call-poly <vilib>:"Number of Waveform Samples.vi"("waveform in"=w258) -> ("number of samples"=w263:i32)  [unwired: 8 in, 2 out]
        n226 = Decrement(x=w263) -> (x-1=w264:i32)
        n227 = To Double Precision Float(number=w264) -> (double precision float=w262:dbl)
        n228 = call-poly <vilib>:"Get Waveform Subset (LV80).vi"("start/duration format"=w261, "duration"=w262, "waveform in"=w258) -> ("waveform out"=w259:waveform(dbl))  [unwired: 3 in, 3 out]
        n229 = Bundle By Name("dt"=w257, "Y"=w259) -> (→"FFT2":waveform(dbl))  [unwired: 1 in]
      }
      frame "Parar" {
      }
      frame "Cálculos" {
        w365 = u16 1 items=["Samples", "Relative Time"] ("start/duration format")
        n230 = local read "Espectro novo"() -> (w351:dbl[])
        n231 = local read "Espectro osso"() -> (w354:dbl[])
        n232 = Array Max & Min(array=w351) -> (max value=w359:dbl, max index (indices)=w358:i32)  [unwired: 2 out]
        n233 = Divide(x=w354, y=w351) -> (x/y=w374:dbl[])
        n234 = Divide(x=w351, y=w359) -> (x/y=w369:dbl[])
        n235 = local read "dfnovo"() -> (w352:dbl)
        n236 = Multiply(x=w352, y=w358) -> (x*y=→"Freq. central":dbl)
        n237 = Logarithm Base 10(1:w374) -> (0:w375:dbl[])
        n238 = Logarithm Base 10(1:w369) -> (0:w370:dbl[])
        n239 = Multiply(x=w375, y=10.0) -> (x*y=w364:dbl[])
        "ABTF" <- w364
        n240 = Multiply(x=w370, y=10.0) -> (x*y=w353:dbl[])
        n241 = local read "Fmin"() -> (w366:dbl)
        n242 = local read "Fmax"() -> (w367:dbl)
        n243 = script code="comeco=min(find(Y>=-6));\nfinal=max(find(Y>=-6));\nF1=df*comeco;\nF2=df*final;\nf = ABTF(comeco:final);\nn = final-comeco;\n% disp(n);\nh = (F2-F1)/(n-1);\nI = 0;\nfor i=1:n-1\nI = I + ((f(i)+f(i+1))/2)*h;\nend\nAIB = I/(F2-F1);" ("Script Node")("Y"=w353, "df"=w352, "ABTF"=w364) -> ("F1"=→"Fmin":dbl, "F2"=→"Fmax":dbl, "AIB"=→"AIB":dbl)  [unwired: 1 in, 1 out]
        n244 = Bundle By Name("dt"=w352, "Y"=w364) -> (w356:waveform(dbl))  [unwired: 1 in]
        n245 = Subtract(x=w367, y=w366) -> (x-y=w368:dbl)
        n246 = call-poly <vilib>:"Get Waveform Subset (LV80).vi"("start/duration format"=w365, "duration"=w368, "start samples/time"=w366, "waveform in"=w356) -> ("waveform out"=w355:waveform(dbl))  [unwired: 2 in, 3 out]
        "ABTF" <- w355
        n247 = call "Curve Fitting"("Signals"=w355) -> ("best fit"=→"FSAB":dynamicdata, "slope"=→"FSAB":dynamicdata)  [unwired: 5 in, 4 out]
      }
      frame "Cálculos2" {
        n248 = local read "Waveform com osso"() -> (w387:waveform(dbl))
        n249 = Unbundle By Name(w387) -> ("Y"=w383:dbl[], "dt"=w384:dbl)
        n250 = Array Size(array=w383) -> (size(s)=w385:i32)
        n251 = for {
          N: 6 -> [_]
          tunnel: w383 -> [w417]
          tunnel: w385 -> [w415]
          tunnel: w384 -> [w408]
          tunnel: [w404] -> w386 mode=indexing
          tunnel: [w402] -> w377 mode=indexing
          i -> [w409]
          w407 = T4 1 items=["Rectangle"=0, "Hanning"=1, "Hamming"=2, "Blackman-Harris"=3, "Exact Blackman"=4, "Blackman"=5, "Flat Top"=6, "4 Term B-Harris "=7, "7 Term B-Harris"=8, "Low Sidelobe"=9, "Blackman Nuttall"=11, "Triangle"=30, "Bartlett-Hanning"=31, "Bohman"=32, "Parzen"=33, "Welch"=34, "Kaiser"=60, "Dolph-Chebyshev"=61, "Gaussian"=62] ("window")
          w416 = u16 0 items=["Samples", "Relative Time"] ("start/duration format")
          n252 = Divide(x=w415, y=6) -> (x/y=w411:dbl)
          n253 = Multiply(x=w409, y=w411) -> (x*y=w413:dbl)
          n254 = Increment(x=w409) -> (x+1=w412:i32)
          n255 = Multiply(x=w412, y=w411) -> (x*y=w403:dbl)
          n256 = call-poly <vilib>:"Get Waveform Subset (LV80).vi"("start/duration format"=w416, "duration"=w403, "start samples/time"=w413, "waveform in"=w417) -> ("waveform out"=w410:waveform(dbl))  [unwired: 2 in, 3 out]
          n257 = Bundle By Name("Y"=w410, "dt"=w408) -> (w406:waveform(dbl))  [unwired: 1 in]
          n258 = call-poly <vilib>:"FFT Power Spectral Density.vi"("window"=w407, "time signal"=w406) -> ("power spectral density"=w405:cluster{"f0":dbl, "df":dbl, "magnitude":dbl[]})  [unwired: 6 in, 3 out]
          n259 = Unbundle By Name(w405) -> ("magnitude"=w404:dbl[], "df"=w402:dbl)
        }
        n260 = while {
          tunnel: [w399] -> w381 mode=indexing
          tunnel: w386 -> [w390] mode=indexing
          tunnel: w377 -> [w389] mode=indexing
          i -> [w394]
          stop <- w393 stop-if-true
          n261 = local read "Espectro novo"() -> (w391:dbl[])
          n262 = Divide(x=w390, y=w391) -> (x/y=w395:dbl[])
          n263 = Equal?(x=5, y=w394) -> (x = y?=w393:bool)
          n264 = Logarithm Base 10(1:w395) -> (0:w397:dbl[])
          n265 = local read "Fmax"() -> (w400:dbl)
          n266 = local read "Fmin"() -> (w401:dbl)
          n267 = Multiply(x=w397, y=10.0) -> (x*y=w396:dbl[])
          n268 = script code="freq=df*(0:size(ABTF,2));\ncomeco=max(find(freq<=F1));\nfinal=min(find(freq>=F2));\nf = ABTF(comeco:final);\nn = final-comeco;\ndisp(n);\nh = (F2-F1)/(n-1);\nI = 0;\nfor i=1:n-1\nI = I + ((f(i)+f(i+1))/2)*h;\nend\nAIB = I/(F2-F1);" ("Script Node")("ABTF"=w396, "F1"=w401, "F2"=w400, "df"=w389) -> ("AIB"=w399:dbl)  [unwired: 1 in, 1 out]
        }
        "AIB's" <- w381
        n269 = call "Convert to Dynamic Data2"("Array"=w381) -> ("Dynamic Data Type"=w380:dynamicdata)  [unwired: 3 in]
        n270 = call "Curve Fitting2"("Signals"=w380) -> ("best fit"=→"TSAB":dynamicdata, "slope"=→"TSAB":dynamicdata)  [unwired: 5 in, 4 out]
      }
      frame "Tabela" {
        n271 = property on="Repetição" class="Ring (strict)"() -> ("Value"=w441:u16)  [unwired: 2 in, 2 out]
        n272 = local read "AIB"() -> (w420:dbl)
        n273 = local read "Tabela de Resultados"() -> (w437:string[][])
        n274 = Increment(x=w441) -> (x+1=w425:u16)
        n275 = Number To Fractional String(use system decimal point (T)=FALSE, number=w420, precision (6)=i16 3) -> (F-format string=w439:string)  [unwired: 1 in]
        n276 = Replace Array Subset(array=w437, new element=w439, index (row)=w425, index (col)=1) -> (w419:string[][])
        n277 = local read "TSAB"() -> (w428:dbl)
        n278 = property on="Repetição" class="Ring (strict)"() -> ("Value"=w429:u16)  [unwired: 2 in, 2 out]
        n279 = Increment(x=w429) -> (x+1=w423:u16)
        n280 = Number To Fractional String(number=w428, precision (6)=i16 3) -> (F-format string=w426:string)  [unwired: 2 in]
        n281 = local read "FSAB"() -> (w433:dbl)
        n282 = Replace Array Subset(array=w419, new element=w426, index (row)=w423, index (col)=3 ("disabled index (col)")) -> (w418:string[][])
        n283 = property on="Repetição" class="Ring (strict)"() -> ("Value"=w434:u16)  [unwired: 2 in, 2 out]
        n284 = Increment(x=w434) -> (x+1=w424:u16)
        n285 = Number To Exponential String(number=w433, precision (6)=i16 3) -> (E-format string=w431:string)  [unwired: 2 in]
        n286 = Replace Array Subset(array=w418, new element=w431, index (row)=w424, index (col)=2 ("disabled index (col)")) -> (w436:string[][])
        n287 = local write "Tabela de Resultados"(w436) -> ()
        n288 = while {
          stop <- w444 stop-if-true
          n289 = One Button Dialog(message="Selecione a repetição na aba \"Configurações\" e clique em \"Run\" ou pressione \"ESC\" para finalizar o programa", button name ("OK")="Ok") -> (true=w444:bool)
        }
      }
      frame "Salvar" {
        n290 = local read "Waveform Referência"() -> (w461:waveform(dbl))
        n291 = local read "Tabela de Resultados"() -> (w455:string[][])
        n292 = local read "Waveform com osso"() -> (w462:waveform(dbl))
        n293 = local read "Observações"() -> (w445:string)
        n294 = local read "ABTF"() -> (w457:waveform(dbl))
        n295 = local read "TSAB"() -> (w456:dynamicdata)
        n296 = local read "Fmax"() -> (w449:dbl)
        n297 = local read "FSAB"() -> (w458:dynamicdata)
        n298 = local read "Fmin"() -> (w450:dbl)
        n299 = local read "FSAB"() -> (w446:dbl)
        n300 = local read "FFT2"() -> (w459:waveform(dbl))
        n301 = local read "AIB's"() -> (w448:dbl[])
        n302 = local read "AIB"() -> (w451:dbl)
        n303 = local read "TSAB"() -> (w447:dbl)
        n304 = local read "FFT1"() -> (w460:waveform(dbl))
        n305 = Bundle("Waveform Referência"=w461, "Waveform com osso"=w462, "FFT1"=w460, "FFT2"=w459, "FSAB"=w458, "ABTF"=w457, "TSAB"=w456, "Tabela de Resultados"=w455, "AIB"=w451, "Fmin"=w450, "Fmax"=w449, "AIB's"=w448, "TSAB"=w447, "FSAB"=w446, "Observações"=w445) -> (w452:T1)  [unwired: 1 in]
        "output cluster" <- w452
        n306 = Write to Binary File(data=w452) -> (refnum out=→"refnum out":refnum<file>)  [unwired: 5 in, 2 out]
      }
      frame "LeituradeDados" {
        w470 = T3."Enabled" ("Disabled")
        n307 = local read "output cluster"() -> (w480:T1)
        n308 = Read from Binary File(5:w480) -> (2:w479:T1)  [unwired: 5 in, 3 out]
        n309 = local write "output cluster"(w479) -> ()
        n310 = Unbundle By Name(w479) -> ("Waveform Referência"=w477:waveform(dbl), "Waveform com osso"=w478:waveform(dbl), "FFT1"=w476:waveform(dbl), "FFT2"=w475:waveform(dbl), "FSAB"=w474:dynamicdata, "ABTF"=w473:waveform(dbl), "TSAB"=w472:dbl, "Tabela de Resultados"=w471:string[][], "AIB"=w469:dbl, "Fmin"=w468:dbl, "Fmax"=w467:dbl, "AIB's"=w466:dbl[], "TSAB"=w465:dynamicdata, "FSAB"=w464:dynamicdata, "Observações"=w463:string)
        n311 = local write "Tabela de Resultados"(w471) -> ()
        n312 = local write "Observações"(w463) -> ()
        n313 = local write "Waveform com osso"(w478) -> ()
        n314 = local write "Waveform Referência"(w477) -> ()
        n315 = local write "TSAB"(w472) -> ()
        n316 = local write "Fmin"(w468) -> ()
        n317 = local write "TSAB"(w465) -> ()
        n318 = local write "FFT1"(w476) -> ()
        n319 = local write "FFT2"(w475) -> ()
        n320 = local write "FSAB"(w474) -> ()
        n321 = local write "ABTF"(w473) -> ()
        n322 = local write "AIB"(w469) -> ()
        n323 = local write "Fmax"(w467) -> ()
        n324 = local write "AIB's"(w466) -> ()
        n325 = local write "FSAB"(w464) -> ()
        n326 = property on="Waveform com osso" class="WFGraph (strict)"("DisabledEnum"=w470) -> ()  [unwired: 2 in, 2 out]
        n327 = property on="Waveform Referência" class="WFGraph (strict)"("DisabledEnum"=w470) -> ()  [unwired: 2 in, 2 out]
        n328 = property on="FFT2" class="WFGraph (strict)"("DisabledEnum"=w470) -> ()  [unwired: 2 in, 2 out]
      }
      frame "Excel" {
        # "Rows"
        n329 = local read "Tabela de Resultados"() -> (w493:string[][])
        n330 = call "Open Excel and Make Visible.vi"("error in (no error)"=errorcluster {"status"=FALSE, "code"=0, "source"=""}, "Visible Boolean"=TRUE) -> ("error out"=w485:errorcluster, "Excel._Application"=w484:refnum<k7>)
        n331 = call "Open New  WorkBook.vi"("error in (no error)"=w485, "Excel._Application"=w484) -> ("error out"=w486:errorcluster, "Excel._Workbook"=w483:refnum<k7>)  [unwired: 1 out]
        n332 = call "Open New WorkSheet.vi"("error in (no error)"=w486, "Excel._Workbook"=w483) -> ("error out"=w482:errorcluster, "Excel._Worksheet"=w481:refnum<k7>)  [unwired: 1 out]
        n333 = Array Size(array=w493) -> (size(s)=w491:i32[])
        n334 = Index Array(array=w491, index=0) -> (element=w489:i32)
        n335 = Index Array(array=w491, index=1) -> (element=w492:i32)
        n336 = for {
          N: w489 -> [_]
          tunnel: w481 -> [w500]
          tunnel: w482 -> [w498]
          tunnel: w493 -> [w497] mode=indexing
          tunnel: w492 -> [w496]
          i -> [w499]
          n337 = for {
            N: w496 -> [_]
            tunnel: w500 -> [w504]
            tunnel: w498 -> [w503]
            tunnel: w499 -> [w502]
            tunnel: w497 -> [w501] mode=indexing
            i -> [w509]
            # "Add Data"
            n338 = Increment(x=w502) -> (x+1=w508:i32)
            n339 = Increment(x=w509) -> (x+1=w506:i32)
            n340 = Increment(x=w508) -> (x+1=w507:i32)
            n341 = Increment(x=w506) -> (x+1=w505:i32)
            n342 = call "Set Cell Value.vi"("Row"=w507, "Col"=w505, "Value"=w501, "error in (no error)"=w503, "Excel._Worksheet"=w504) -> ()  [unwired: 2 out]
          }
        }
      }
    }
    n343 = Or(x=w4, y=w3) -> (x .or. y?=w2:bool)
  }
